vi "UtilityLib.set color of simple string or numeric.vi"(0 "simpleString":refnum<vi>, 1 "simpleNumeric":refnum<vi>, 2 "valueStatus":T1, 5 "error in (no error)":errorcluster) -> (19 "error out":errorcluster)   [LabVIEW 2014, in "UtilityLib.lvlib"]
doc: "Set the color of a SIMPLE (classic control) text or numeric control/indicator to a value defined in six-color vi."
uses:
  UtilityLib.lvlib
  UtilityLib.valueStatus.ctl
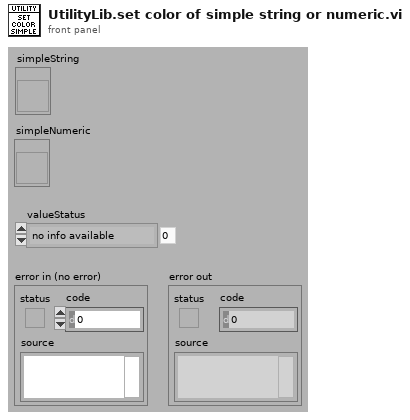
[diagram p1: front panel]
types:
  T1 = typedef "UtilityLib.lvlib/UtilityLib.valueStatus.ctl" = enum16{"no info available", "stand by/off", "on", "warning", "alarm/malfunction", "not implemented", "user action required", "important information", "system default", "control default", "indicator default", "button default"}
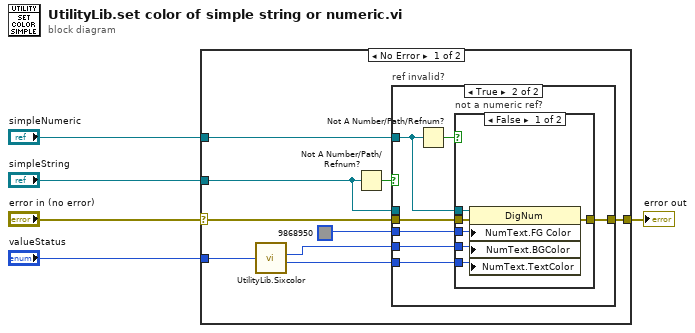
[diagram p0: block diagram]
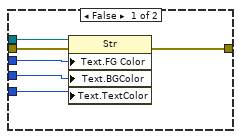
[diagram p2: hidden frame]
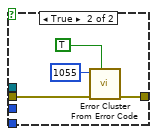
[diagram p3: hidden frame]
diagram:
  n1 = case shown="No Error" "error in (no error)" {
    selector: "error in (no error)" -> [w6 w38]
    tunnel: [w14 w38] -> w5
    tunnel: "simpleString" -> [w13 _]
    tunnel: "simpleNumeric" -> [w8 _]
    tunnel: "valueStatus" -> [w7 _]
    frame No Error {
      n2 = call "UtilityLib.Sixcolor.vi"("State"=w7) -> ("elementBackground"=w11:u32, "elementText"=w10:u32)  [unwired: 2 in, 2 out]
      n3 = Not A Number/Path/Refnum?(number/path/refnum=w13) -> (NaN/Path/Refnum?=w9:bool)
      n4 = case "ref invalid?" shown="True" w9 {
        tunnel: [w20 w27] -> w14
        tunnel: w6 -> [w19 w26]
        tunnel: w13 -> [w18 _]
        tunnel: u32 9868950 ("Color Box") -> [w17 w25]
        tunnel: w11 -> [w16 w24]
        tunnel: w10 -> [w15 w23]
        tunnel: w8 -> [_ w22]
        frame False {
          n5 = property class="Str"(reference=w18, error in=w19, "Text.FG Color"=w17, "Text.BGColor"=w16, "Text.TextColor"=w15) -> (error out=w20:errorcluster)  [unwired: 1 out]
        }
        frame True {
          n6 = Not A Number/Path/Refnum?(number/path/refnum=w22) -> (NaN/Path/Refnum?=w21:bool)
          n7 = case "not a numeric ref?" shown="False" w21 {
            tunnel: [w33 w36] -> w27
            tunnel: w26 -> [w32 w37]
            tunnel: w25 -> [w31 _]
            tunnel: w24 -> [w30 _]
            tunnel: w23 -> [w29 _]
            tunnel: w22 -> [w28 _]
            frame False {
              n8 = property class="DigNum"(reference=w28, error in=w32, "NumText.FG Color"=w31, "NumText.BGColor"=w30, "NumText.TextColor"=w29) -> (error out=w33:errorcluster)  [unwired: 1 out]
            }
            frame True {
              n9 = call <vilib>:"Error Cluster From Error Code.vi"("show call chain? (False)"=TRUE, "error in (no error)"=w37, "error code (0)"=1055) -> ("error out"=w36:errorcluster)  [unwired: 6 in]
            }
          }
        }
      }
    }
    frame Error {
    }
  }
  "error out" <- w5
